vi "simple.vi"() -> (3 "Numeric":i32)   [LabVIEW 2013]
uses:
  XControl.xctl
panel:
  in  "XControl":dbl(xcontrol)
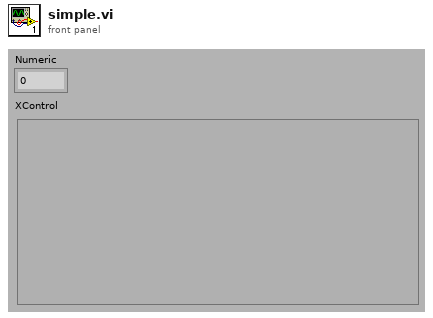
[diagram p1: front panel]
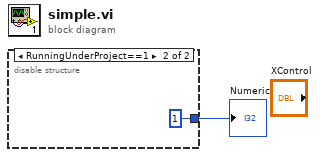
[diagram p0: block diagram]
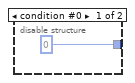
[diagram p2: hidden frame]
diagram:
  n1 = disable-structure shown="RunningUnderProject==1" {
    disable-tunnel: [0 1 ("Numeric")] -> w1
    frame condition #0 {
    }
    frame condition #1 (active) {
    }
  }
  "Numeric" <- w1
